vi "DiffDrivePoseEst_BiFunc_H.vi"(9 "U":T1, 10 "X":T1, 11 "ExtraPassedData":variant) -> (0 "Error":bool, 3 "Result":T1)   [LabVIEW 2019, in "Trajectory_Library.lvlib"]
doc: "H function to pass to kalmanfilter correct."
uses:
  Trajectory_Library.lvlib
  <vilib>/Analysis/Matrix/Datatypes/RealMatrix.ctl
  MatBuilder_Create.vi
  <vilib>/Analysis/Matrix/NI_Matrix.lvlib
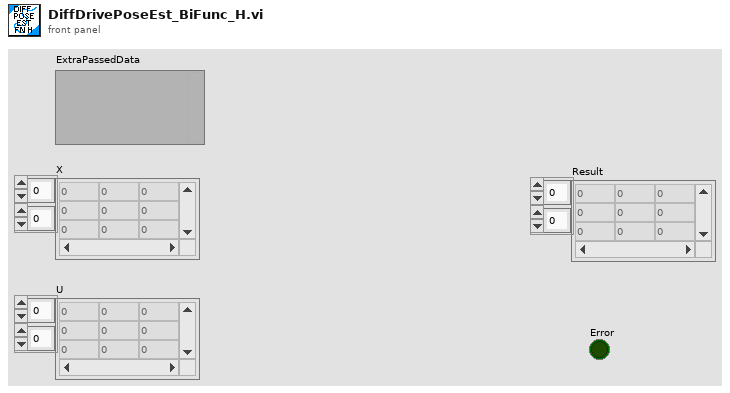
[diagram p1: front panel]
types:
  T1 = typedef "NI_Matrix.lvlib/RealMatrix.ctl" = dbl[][]
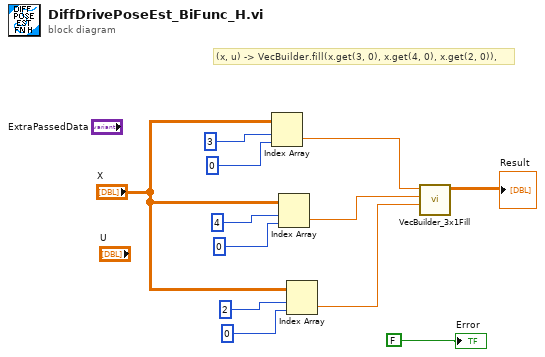
[diagram p0: block diagram]
diagram:
  # "(x, u) -> VecBuilder.fill(x.get(3, 0), x.get(4, 0), x.get(2, 0)),"
  n1 = Index Array(array="X", index (row)=3, index (col)=0) -> (element=w4:dbl)
  n2 = Index Array(array="X", index (row)=4, index (col)=0) -> (element=w3:dbl)
  n3 = Index Array(array="X", index (row)=2, index (col)=0) -> (element=w2:dbl)
  n4 = call "VecBuilder_3x1Fill.vi"("R2"=w2, "R1"=w3, "R0"=w4) -> ("output matrix"=→"Result":T1)  [unwired: 8 in]
  "Error" <- FALSE
